vi "Tablet.vi"() -> ()   [LabVIEW 2011]
panel:
  out "Waveform Graph":dbl[](graph)
  in  "Slide":dbl(slide) scale=0.0..10.0
  in  "Boolean":bool
  out "Running":bool
  in  "Channel":u16(ring) items=["one", "two", "three"]
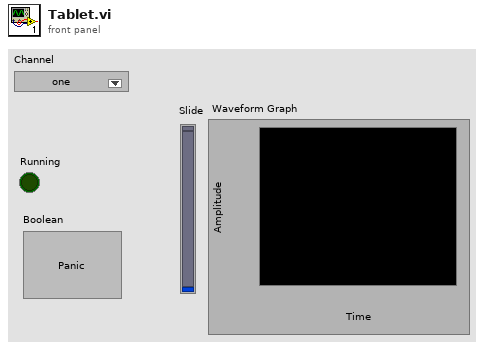
[diagram p1: front panel]
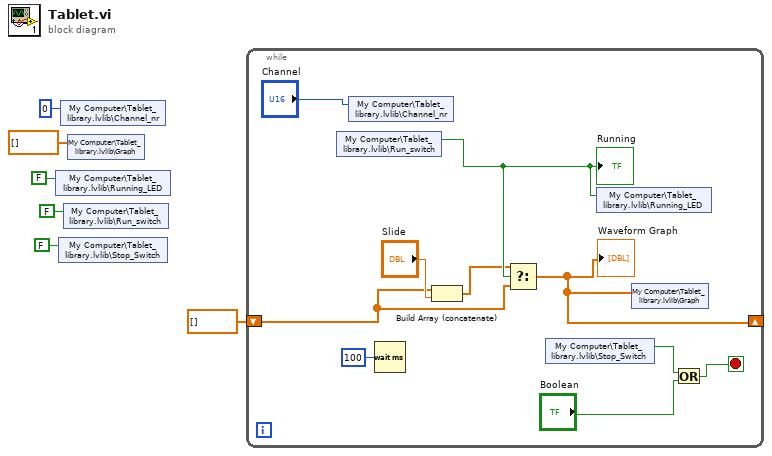
[diagram p0: block diagram]
diagram:
  n1 = shared-variable "My Computer\\Tablet_library.lvlib\\Running_LED"(FALSE ("Running_LED")) -> ()  [unwired: 1 in, 1 out]
  n2 = shared-variable "My Computer\\Tablet_library.lvlib\\Stop_Switch"(FALSE ("Stop_Switch")) -> ()  [unwired: 1 in, 1 out]
  n3 = shared-variable "My Computer\\Tablet_library.lvlib\\Channel_nr"(0 ("Channel_nr")) -> ()  [unwired: 1 in, 1 out]
  n4 = shared-variable "My Computer\\Tablet_library.lvlib\\Run_switch"(FALSE ("start_switch")) -> ()  [unwired: 1 in, 1 out]
  n5 = shared-variable "My Computer\\Tablet_library.lvlib\\Graph"(dbl[] [] ("Graph")) -> ()  [unwired: 1 in, 1 out]
  n6 = while {
    shift-right: [w9] -> _
    shift-left: dbl[] [] -> [w8]
    stop <- w12 stop-if-true
    n7 = shared-variable "My Computer\\Tablet_library.lvlib\\Run_switch"() -> (w11:bool)  [unwired: 1 in, 1 out]
    "Running" <- w11
    n8 = shared-variable "My Computer\\Tablet_library.lvlib\\Channel_nr"("Channel") -> ()  [unwired: 1 in, 1 out]
    n9 = Wait (ms)(milliseconds to wait=u32 100) -> ()  [unwired: 1 out]
    n10 = Build Array (concatenate)(w8, "Slide") -> (w10:dbl[])
    n11 = Select(t=w10, s=w11, f=w8) -> (s? t:f=w9:dbl[])
    "Waveform Graph" <- w9
    n12 = shared-variable "My Computer\\Tablet_library.lvlib\\Stop_Switch"() -> (w13:bool)  [unwired: 1 in, 1 out]
    n13 = shared-variable "My Computer\\Tablet_library.lvlib\\Running_LED"(w11) -> ()  [unwired: 1 in, 1 out]
    n14 = shared-variable "My Computer\\Tablet_library.lvlib\\Graph"(w9) -> ()  [unwired: 1 in, 1 out]
    n15 = Or(x=w13, y="Boolean") -> (x .or. y?=w12:bool)
  }
